vi "Check Session Properties.vi"(0 "VISA resource name":refnum<visa-resource-name>, 11 "error in (no error)":errorcluster) -> (3 "Model 6485":bool, 4 "VISA resource name out":refnum<visa-resource-name>, 8 "Interface Type":u16(ring)=1 items=["GPIB"=1, "VXI"=2, "GPIB-VXI"=3, "Serial"=4, "PXI"=5, "TCPIP"=6, "USB"=7, "FireWire"=9], 15 "error out":errorcluster)   [LabVIEW 2020, in "Keithley 648X Series.lvlib"]
doc: "Get the interface type and model."
uses:
  <instrlib>/Keithley 648X Series/Keithley 648X Series.lvlib
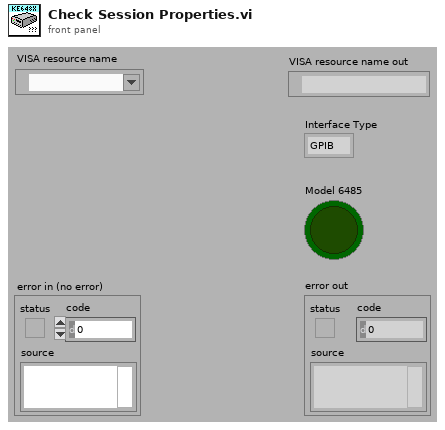
[diagram p1: front panel]
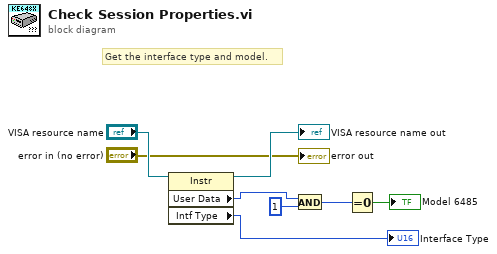
[diagram p0: block diagram]
diagram:
  # "Get the interface type and model."
  n1 = property class="Instr"(reference="VISA resource name") -> (reference out=→"VISA resource name out":refnum<visa-resource-name>, "User Data"=w5:u32, "Intf Type"=→"Interface Type":u16)  [unwired: 1 in, 1 out]
  n2 = And(x=w5, y=u32 1) -> (x .and. y?=w3:u32)
  n3 = Equal To 0?(x=w3) -> (x = 0?=→"Model 6485":bool)
  "error out" <- "error in (no error)"
